vi "DRIVE_STOP.vi"(10 "argv":string[](array[string]), 11 "args":u8) -> ()   [LabVIEW 2011]
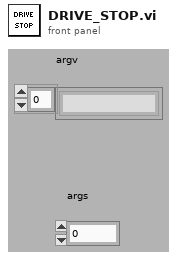
[diagram p1: front panel]
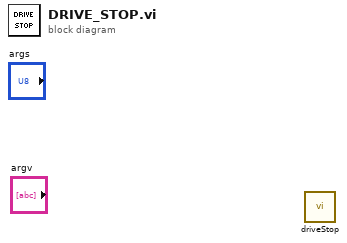
[diagram p0: block diagram]
diagram:
  n1 = call "driveStop.vi"() -> ()  [unwired: 12 in]
